vi "Create HTTP Session.vi"(8 "error in (no error)":errorcluster, 10 "Username":string, 11 "Web Request in":refnum<class "Web Request.lvclass">) -> (0 "error out":errorcluster, 3 "Web Request out":refnum<class "Web Request.lvclass">)   [LabVIEW 2016, in "WSsupport.lvlib"]
uses:
  WSsupport.lvlib
  <vilib>/wsapi/Web Request.lvclass
  <vilib>/wsapi/class/subVIs/Write Single Session Variable.vi
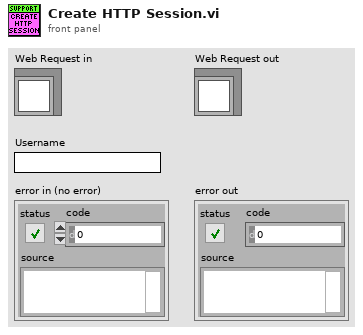
[diagram p1: front panel]
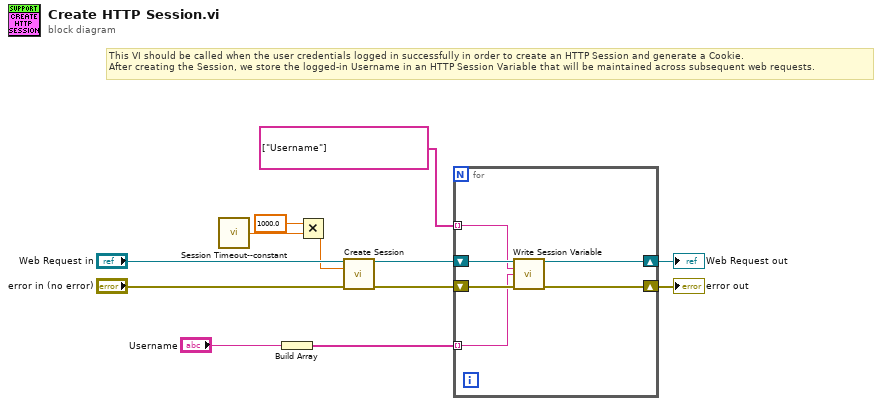
[diagram p0: block diagram]
diagram:
  # "This VI should be called when the user credentials logged in successfully in order to create an HTTP Session and generate a Cookie.\nAfter creating the Session, we store the logged-in Username in an HTTP Session Variable that will be maintained across subsequent web requests."
  n1 = call "Session Timeout--constant.vi"() -> ("Session Timeout (s)"=w7:dbl)
  n2 = Build Array("Username") -> (w4:string[])
  n3 = Multiply(x=1000.0, y=w7) -> (x*y=w6:dbl)
  n4 = call <vilib>:"Create Session.vi"("LabVIEW Web Service Request"="Web Request in", "timeout (60000 msec)"=w6, "error in (no error)"="error in (no error)") -> ("LabVIEW Web Service Request out"=w9:refnum<class "Web Request.lvclass">, "error out"=w8:errorcluster)  [unwired: 10 in, 1 out]
  n5 = for {
    shift-right: [w17] -> w11
    shift-left: w9 -> [w16]
    shift-right: [w18] -> w12
    shift-left: w8 -> [w15]
    tunnel: w4 -> [w14] mode=indexing
    tunnel: string[] ["Username"] -> [w13] mode=indexing
    n6 = call-poly <vilib>:"Write Session Variable.vi"("LabVIEW Web Service Request"=w16, "key"=w13, "value"=w14, "error in (no error)"=w15) -> ("LabVIEW Web Service Request out"=w17:refnum<class "Web Request.lvclass">, "error out"=w18:errorcluster)  [unwired: 8 in, 2 out]
  }
  "error out" <- w12
  "Web Request out" <- w11
